vi "MtAtElectrometer_registerCallback_command_stopScanackcmd.vi"(8 "error in (no error)":errorcluster, 10 "skipOld":bool, 11 "handle":i32) -> (0 "error out":errorcluster, 3 "function return":i32)   [LabVIEW 2016, in "SALLV_MtAtElectrometer.lvlib"]
doc: "int MtAtElectrometer_shm_registerCallback_command_stopScan_ackcmdLV(int handle, bool skipOld);"
uses:
  SALLV_MtAtElectrometer.lvlib
  ts_sal/test/MtAtElectrometer/labview/SALLV_MtAtElectrometer.so
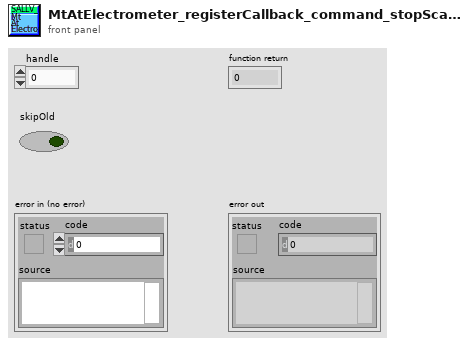
[diagram p1: front panel]
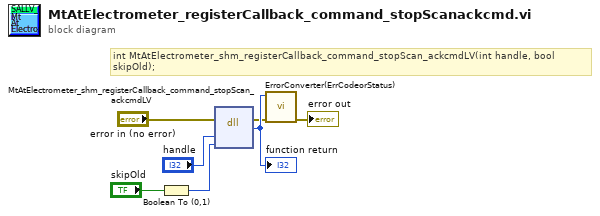
[diagram p0: block diagram]
diagram:
  # "int MtAtElectrometer_shm_registerCallback_command_stopScan_ackcmdLV(int handle, bool skipOld);"
  n1 = Boolean To (0,1)(Boolean="skipOld") -> (0, 1=w4:i16)
  n2 = dll-call lib="home/andres/ts_sal/test/MtAtElectrometer/labview/SALLV_MtAtElectrometer.*" fn="MtAtElectrometer_shm_registerCallback_command_stopScan_ackcmdLV"(error in="error in (no error)", "handle"="handle", "skipOld"=w4) -> (error out=w2:errorcluster, w7:i32)  [unwired: 4 in, 1 out]
  "function return" <- w7
  n3 = call "ErrorConverter(ErrCodeorStatus).vi"("error in (no error)"=w2, "error code"=w7) -> ("error out"=→"error out":errorcluster)  [unwired: 9 in]
